vi "FGV GD Status Anzeige.vi"(6 "Aktion":T1, 7 "aufsteigend":bool, 8 "error in (no error)":errorcluster caption="Fehler (Eingang, kein Fehler)", 11 "Zustand in":string) -> (0 "error out":errorcluster caption="Fehler (Ausgang)", 3 "Zustand out":string)   [LabVIEW 2020, in "Linearisierung v2.lvlib"]
uses:
  Linearisierung v2.lvlib
  Aktion FGV GD Status Anzeige.ctl
  Allgemein/allgemeine Sub-VIs.lvlib
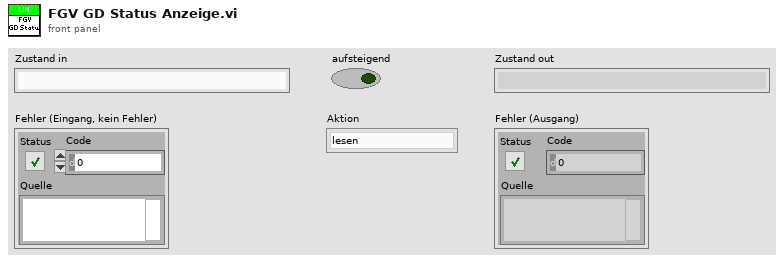
[diagram p1: front panel]
types:
  T1 = typedef "Linearisierung v2.lvlib/Aktion FGV GD Status Anzeige.ctl" = enum16{"lesen", "schreiben", "hinzufügen"}
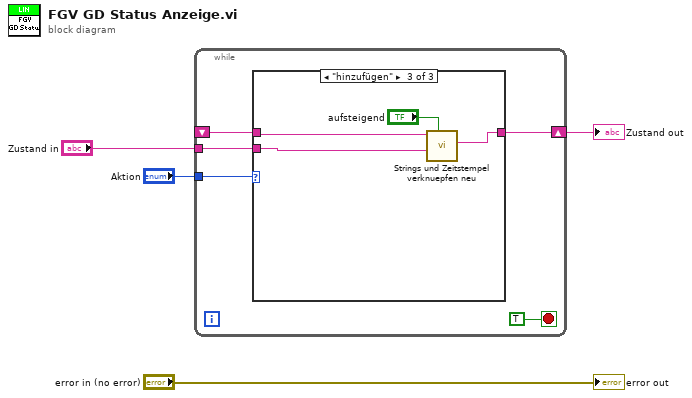
[diagram p0: block diagram]
diagram:
  n1 = while {
    tunnel: "Aktion" -> [w9]
    shift-right: [w7] -> w3
    shift-left: _ -> [w6]
    tunnel: "Zustand in" -> [w5]
    stop <- TRUE stop-if-true
    n2 = case shown="\"hinzufügen\"" w9 {
      tunnel: [w10 w11 w12] -> w7
      tunnel: w6 -> [w10 _ w14]
      tunnel: w5 -> [_ w11 w13]
      frame "lesen", Default {
      }
      frame "schreiben" {
      }
      frame "hinzufügen" {
        n3 = call "Strings und Zeitstempel verknuepfen neu.vi"("aufsteigend"="aufsteigend", "String 1 hinzufügen"=w13, "Eingangs String"=w14) -> ("Verknüpfter String"=w12:string)  [unwired: 8 in]
      }
    }
  }
  "Zustand out" <- w3
  "error out" <- "error in (no error)"
